vi "DC Basic Configure.vi"(0 "Channel 2":bool, 3 "Channel 1":bool=TRUE, 4 "Voltmeter Buffer Size":string="22", 5 "Voltmeter 2 Address":string="11", 6 "Voltmeter Range (V)":string="0.01", 7 "Voltmeter 1 Address":string="7", 8 "NPLC":string="1", 9 "INIT Wave":bool, 10 "Current Amplitude":string="1e-6", 11 "6221 Address":string="12") -> ()   [LabVIEW 2020]
panel:
  out "2182A Input Command":string="*RST\n:SYSTem:AZERo:STATe OFF\n:SENSe:VOLTage:DC:LPASs OFF\n:SENSe:VOLTage:DC:DFILter OFF\n:SENSe:VOLTage:DC:RANGe 0.01\n:form:elem read, tst\n:disp:enab ON\n:sens:volt:nplc 1\n:trig:sour imm\n:init:cont off\n:abort\n:trac:clear\n:trac:poin 82\n:trac:feed sens\n:trac:feed:cont next"
  out "6221 Commands":string="*RST\nOUTPUT:LTEARTH ON\nCLEar\nCURRent:RANGe:AUTO ON\nCURRent:COMPliance 50\nCURRent 1e-6\n"
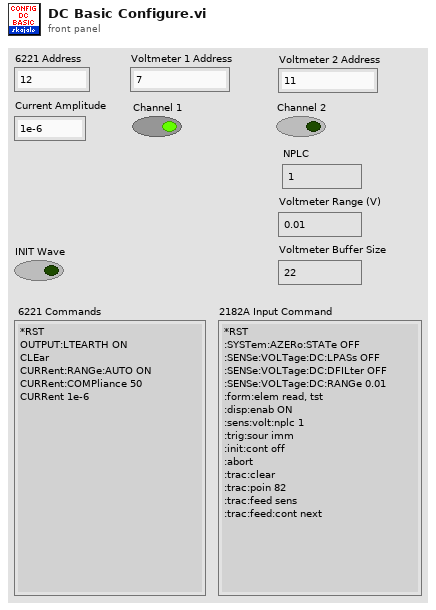
[diagram p1: front panel]
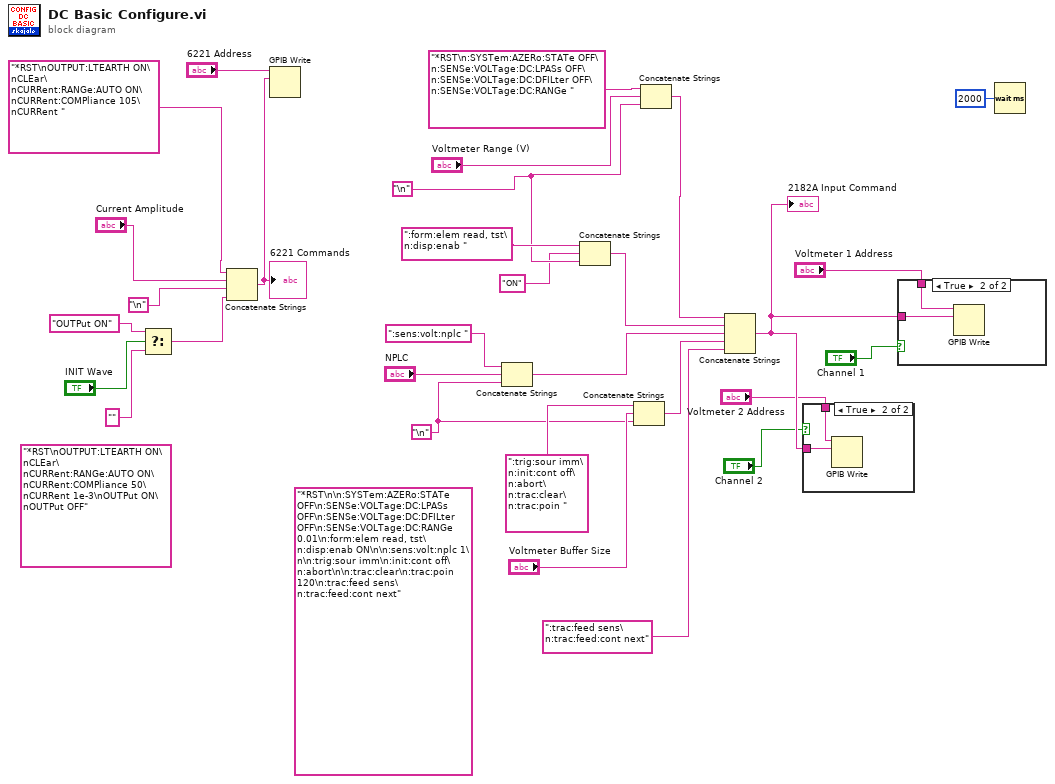
[diagram p0: block diagram]
diagram:
  w11 = "\n"
  (unwired) "*RST\n\n:SYSTem:AZERo:STATe OFF\n:SENSe:VOLTage:DC:LPASs OFF\n:SENSe:VOLTage:DC:DFILter OFF\n:SENSe:VOLTage:DC:RANGe 0.01\n:form:elem read, tst\n:disp:enab ON\n\n:sens:volt:nplc 1\n\n:trig:sour imm\n:init:cont off\n:abort\n\n:trac:clear\n:trac:poin 120\n:trac:feed sens\n:trac:feed:cont next"
  w13 = "\n"
  (unwired) "*RST\nOUTPUT:LTEARTH ON\nCLEar\nCURRent:RANGe:AUTO ON\nCURRent:COMPliance 50\nCURRent 1e-3\nOUTPut ON\nOUTPut OFF" ("data")
  n1 = Select(t="OUTPut ON" ("string"), s="INIT Wave", f="" ("string")) -> (s? t:f=w27:string)
  n2 = Concatenate Strings("*RST\nOUTPUT:LTEARTH ON\nCLEar\nCURRent:RANGe:AUTO ON\nCURRent:COMPliance 105\nCURRent ", "Current Amplitude", "\n", w27) -> (w29:string)
  "6221 Commands" <- w29
  n3 = GPIB Write(0:"6221 Address", 1:w29) -> ()  [unwired: 3 in, 2 out]
  n4 = Concatenate Strings(":sens:volt:nplc ", "NPLC", w11) -> (w16:string)
  n5 = Concatenate Strings(":form:elem read, tst\n:disp:enab ", "ON" ("string"), w13) -> (w17:string)
  n6 = Concatenate Strings(":trig:sour imm\n:init:cont off\n:abort\n:trac:clear\n:trac:poin ", "Voltmeter Buffer Size", w11) -> (w15:string)
  n7 = Concatenate Strings("*RST\n:SYSTem:AZERo:STATe OFF\n:SENSe:VOLTage:DC:LPASs OFF\n:SENSe:VOLTage:DC:DFILter OFF\n:SENSe:VOLTage:DC:RANGe ", "Voltmeter Range (V)", w13) -> (w18:string)
  n8 = Concatenate Strings(w18, w17, w16, w15, ":trac:feed sens\n:trac:feed:cont next") -> (w9:string)
  "2182A Input Command" <- w9
  n9 = case shown="True" "Channel 2" {
    tunnel: w9 -> [_ w32]
    tunnel: "Voltmeter 2 Address" -> [_ w31]
    frame False {
    }
    frame True {
      n10 = GPIB Write(0:w31, 1:w32) -> ()  [unwired: 3 in, 2 out]
    }
  }
  n11 = case shown="True" "Channel 1" {
    tunnel: "Voltmeter 1 Address" -> [_ w34]
    tunnel: w9 -> [_ w33]
    frame False {
    }
    frame True {
      n12 = GPIB Write(0:w34, 1:w33) -> ()  [unwired: 3 in, 2 out]
    }
  }
  n13 = Wait (ms)(milliseconds to wait=u32 2000) -> ()  [unwired: 1 out]
